vi "AccerlationAndSkidpadMonitoring.vi"() -> ()   [LabVIEW 2017]
uses:
  Control/AccelerationIndicator(Monitoring).ctl
  Control/SkidpadIndicator(Monitoring).ctl
  Control/AccelerationBestIndicator(Monitoring).ctl
  Control/AccerlationData.ctl
  Control/SkidpadData.ctl
panel:
  out "SkidpadBestIndicator":T1
  out "AccelerationBestIndicator":T1
  in  "Stop Button":bool
  out "SkidpadIndicator":T2
  out "AccelerationIndicator":T3
  # "2018 KSAE Formula Accerlation & Skidpad Event"
  # "Lap2 :"
  # "Lap4 :"
  # "Total :"
  # "Entry :"
  # "Univ. :"
  # "Time :"
  # "Entry :"
  # "Univ. :"
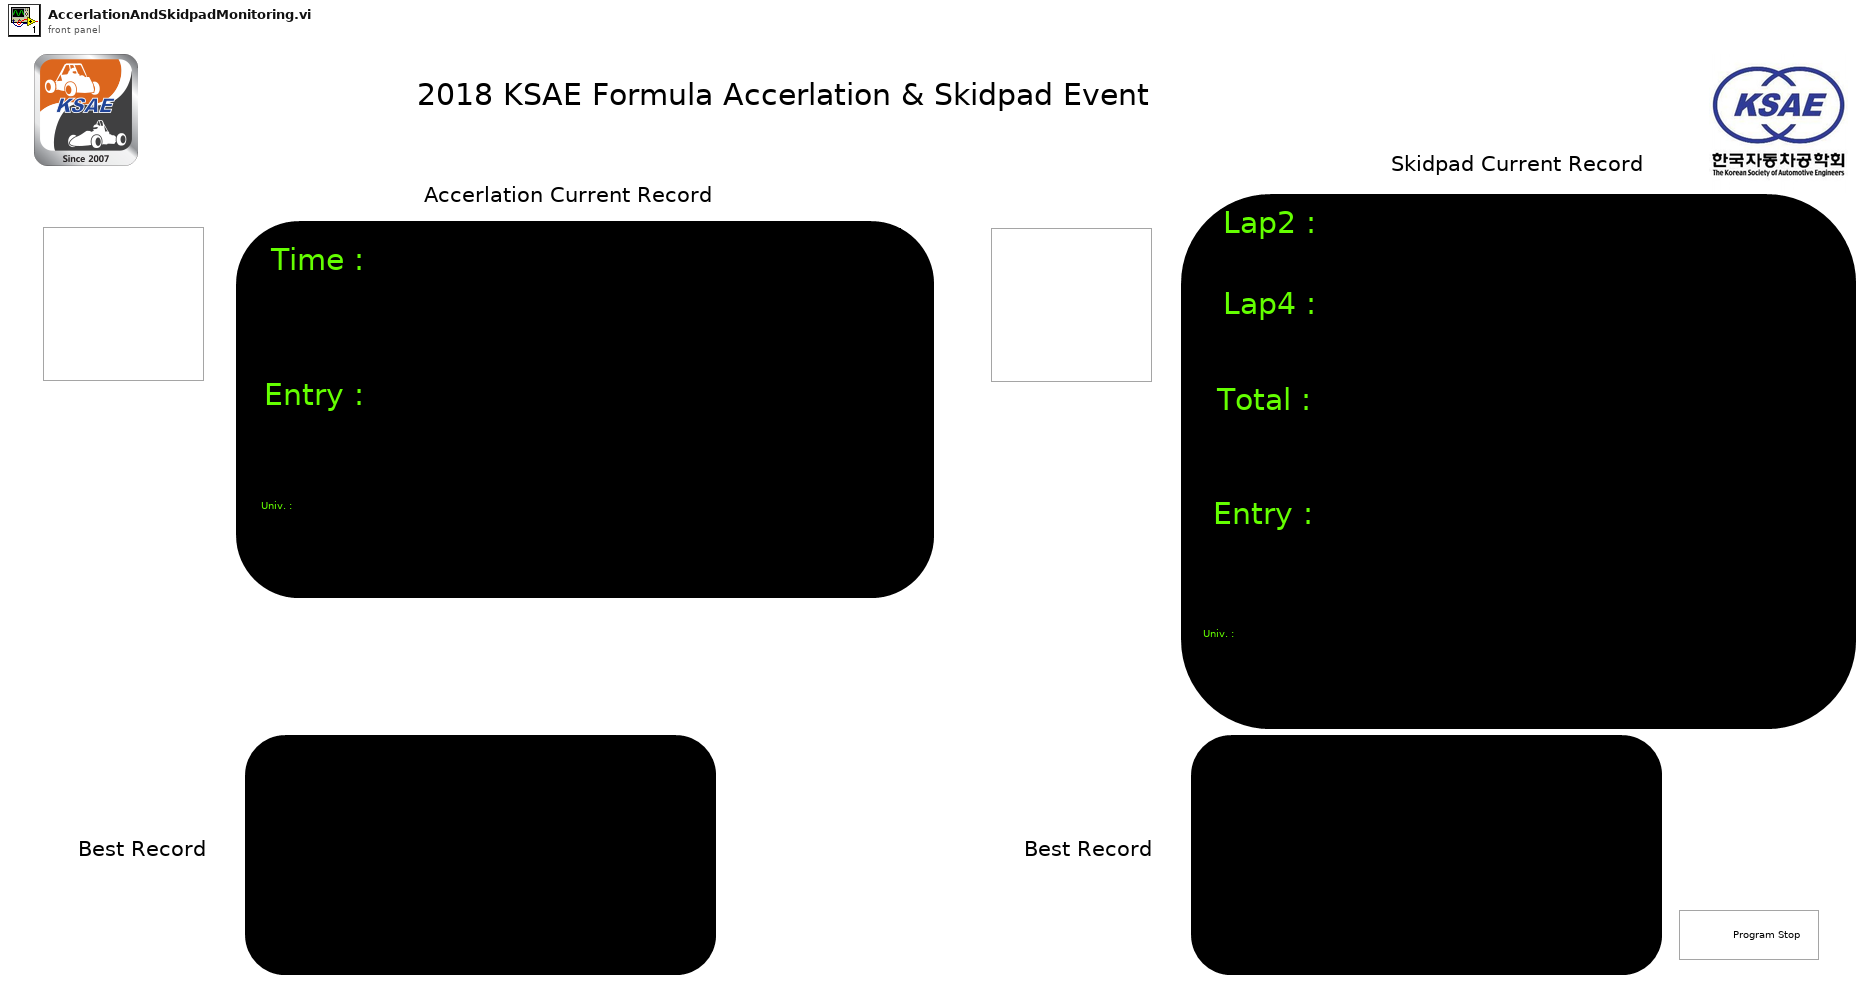
[diagram p1: front panel]
types:
  T1 = typedef "AccelerationBestIndicator(Monitoring).ctl" = cluster{"BestTime":string, "BestEntry":string, "BestSchool":string}
  T2 = typedef "SkidpadIndicator(Monitoring).ctl" = cluster{"Lab2":string, "Lab4":string, "TotalLabTime":string, "CurrentEntry":string, "CurrentSchool":string, "Flag":picture, "CurrentState":string}
  T3 = typedef "AccelerationIndicator(Monitoring).ctl" = cluster{"CurrentTime":string, "CurrentEntry":string, "CurrentUniversity":string, "Flag":picture, "CurrentState":string}
  T4 = typedef "SkidpadData.ctl" = cluster{"LabTime-2":string, "LabTime-4":string, "TotalLabTime":string, "Entry":string, "University":string, "Flag":picture, "Message":string, "TotalLabTimeBest":string, "EntryBest":string, "UniversityBest":string}
  T5 = cluster{"Read Access":enum8{"Allowed", "Required", "None"}, "Write Access":enum8{"Allowed", "Required", "None"}}
  T6 = typedef "AccerlationData.ctl" = cluster{"LabTimeCurrent":string, "EntryCurrent":string, "UniversityCurrent":string, "Flag":picture, "Message":string, "LabTimeBest":string, "EntryBest":string, "UniversityBest":string}
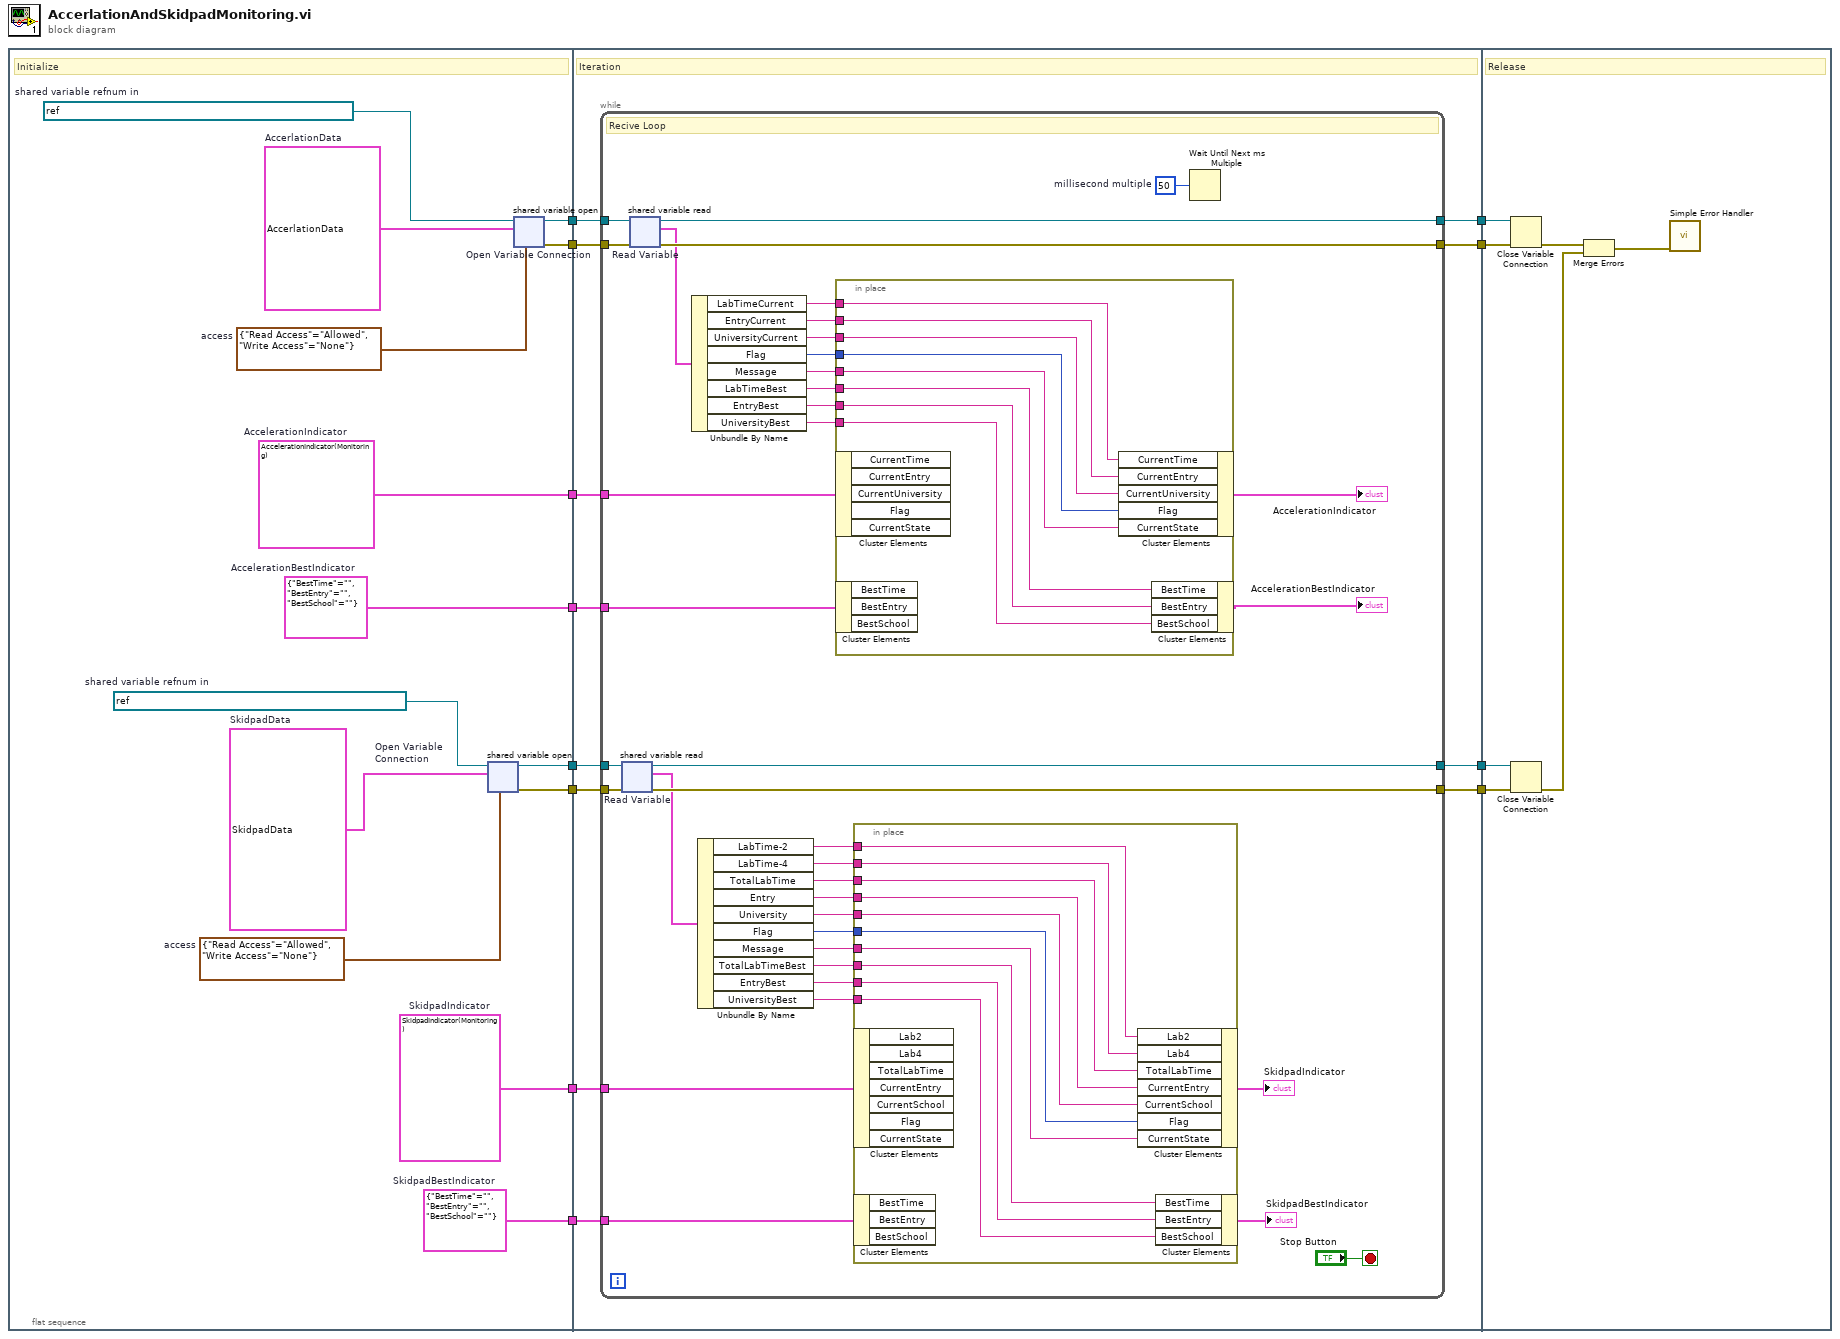
[diagram p0: block diagram]
diagram:
  n1 = flat-sequence {
    tunnel: [w25] -> w12
    tunnel: [w23] -> w11
    tunnel: [w20] -> w8
    tunnel: [w19] -> w7
    tunnel: [w17] -> w4
    tunnel: [w16] -> w3
    tunnel: [w15] -> w2
    tunnel: [w13] -> w1
    tunnel: w12 -> [w38]
    tunnel: w11 -> [w37]
    tunnel: [w36] -> w10
    tunnel: [w35] -> w9
    tunnel: w8 -> [w34]
    tunnel: w7 -> [w33]
    tunnel: [w32] -> w6
    tunnel: [w31] -> w5
    tunnel: w4 -> [w30]
    tunnel: w3 -> [w29]
    tunnel: w2 -> [w28]
    tunnel: w1 -> [w27]
    tunnel: w10 -> [w101]
    tunnel: w9 -> [w100]
    tunnel: w6 -> [w98]
    tunnel: w5 -> [w97]
    frame #0 {
      w13 = T1 {"BestTime"="", "BestEntry"="", "BestSchool"=""}  # SkidpadBestIndicator
      w14 = T4 {"LabTime-2"="", "LabTime-4"="", "TotalLabTime"="", "Entry"="", "University"="", "Flag"=bytes[0], "Message"="", "TotalLabTimeBest"="", "EntryBest"="", "UniversityBest"=""}  # SkidpadData
      w15 = T1 {"BestTime"="", "BestEntry"="", "BestSchool"=""}  # AccelerationBestIndicator
      w16 = T2 {"Lab2"="", "Lab4"="", "TotalLabTime"="", "CurrentEntry"="", "CurrentSchool"="", "Flag"=bytes[0], "CurrentState"=""}  # SkidpadIndicator
      w17 = T3 {"CurrentTime"="", "CurrentEntry"="", "CurrentUniversity"="", "Flag"=bytes[0], "CurrentState"=""}  # AccelerationIndicator
      w18 = refnum<k21> "ni.var.psp://kdh/MonitoringVariable/SkidpadData"  # shared variable refnum in
      w21 = T5 {"Read Access"=enum."Allowed", "Write Access"=enum."None"}  # access
      w22 = refnum<k21> "ni.var.psp://kdh/MonitoringVariable/AccerlationData"  # shared variable refnum in
      w24 = T5 {"Read Access"=enum."Allowed", "Write Access"=enum."None"}  # access
      w26 = T6 {"LabTimeCurrent"="", "EntryCurrent"="", "UniversityCurrent"="", "Flag"=bytes[0], "Message"="", "LabTimeBest"="", "EntryBest"="", "UniversityBest"=""}  # AccerlationData
      # "Initialize"
      n2 = shared-variable-open "Open Variable Connection"(w18, w14, w21) -> (w20:refnum<k21>, w19:errorcluster)  [unwired: 1 in]
      n3 = shared-variable-open "Open Variable Connection"(w22, w26, w24) -> (w25:refnum<k21>, w23:errorcluster)  [unwired: 1 in]
    }
    frame #1 {
      # "Iteration"
      n4 = while {
        tunnel: w38 -> [w76]
        tunnel: w37 -> [w75]
        tunnel: [w73] -> w35
        tunnel: [w72] -> w36
        tunnel: w34 -> [w70]
        tunnel: w33 -> [w69]
        tunnel: [w68] -> w32
        tunnel: [w67] -> w31
        tunnel: w30 -> [w65]
        tunnel: w29 -> [w58]
        tunnel: w28 -> [w48]
        tunnel: w27 -> [w43]
        stop <- "Stop Button" stop-if-true
        w74 = u32 50  # millisecond multiple
        # "Recive Loop"
        n5 = shared-variable-read "Read Variable"(w70, w69) -> (w68:refnum<k21>, w67:errorcluster, w66:T4)  [unwired: 1 out]
        n6 = shared-variable-read "Read Variable"(w76, w75) -> (w73:refnum<k21>, w72:errorcluster, w71:T6)  [unwired: 1 out]
        n7 = Unbundle By Name(w71) -> ("LabTimeCurrent"=w63:string, "EntryCurrent"=w62:string, "UniversityCurrent"=w61:string, "Flag"=w60:picture, "Message"=w59:string, "LabTimeBest"=w47:string, "EntryBest"=w46:string, "UniversityBest"=w45:string)
        n8 = Unbundle By Name(w66) -> ("LabTime-2"=w57:string, "LabTime-4"=w56:string, "TotalLabTime"=w55:string, "Entry"=w54:string, "University"=w52:string, "Flag"=w51:picture, "Message"=w50:string, "TotalLabTimeBest"=w42:string, "EntryBest"=w41:string, "UniversityBest"=w40:string)
        n9 = in-place {
          in-place-border: w63 -> [w94]
          in-place-border: w62 -> [w93]
          in-place-border: w61 -> [w92]
          in-place-border: w60 -> [w91]
          in-place-border: w59 -> [w90]
          in-place-border: w47 -> [w89]
          in-place-border: w46 -> [w88]
          in-place-border: w45 -> [w87]
          n10 = in-place-cluster #1(w65) -> ()  [unwired: 5 out]
          n11 = in-place-cluster #2(w48) -> ()  [unwired: 3 out]
          n12 = in-place-cluster #1("CurrentTime"=w94, "CurrentEntry"=w93, "CurrentUniversity"=w92, "Flag"=w91, "CurrentState"=w90) -> (→"AccelerationIndicator":T3)
          n13 = in-place-cluster #2("BestTime"=w89, "BestEntry"=w88, "BestSchool"=w87) -> (→"AccelerationBestIndicator":T1)
        }
        n14 = in-place {
          in-place-border: w57 -> [w86]
          in-place-border: w56 -> [w85]
          in-place-border: w55 -> [w84]
          in-place-border: w54 -> [w83]
          in-place-border: w52 -> [w82]
          in-place-border: w51 -> [w81]
          in-place-border: w50 -> [w80]
          in-place-border: w42 -> [w79]
          in-place-border: w41 -> [w78]
          in-place-border: w40 -> [w77]
          n15 = in-place-cluster #3(w58) -> ()  [unwired: 7 out]
          n16 = in-place-cluster #4(w43) -> ()  [unwired: 3 out]
          n17 = in-place-cluster #3("Lab2"=w86, "Lab4"=w85, "TotalLabTime"=w84, "CurrentEntry"=w83, "CurrentSchool"=w82, "Flag"=w81, "CurrentState"=w80) -> (→"SkidpadIndicator":T2)
          n18 = in-place-cluster #4("BestTime"=w79, "BestEntry"=w78, "BestSchool"=w77) -> (→"SkidpadBestIndicator":T1)
        }
        n19 = Wait Until Next ms Multiple(millisecond multiple=w74) -> ()  [unwired: 1 out]
      }
    }
    frame #2 {
      # "Release"
      n20 = Close Variable Connection(8:w101, 11:w100) -> (0:w99:errorcluster)
      n21 = Close Variable Connection(8:w97, 11:w98) -> (0:w95:errorcluster)
      n22 = Merge Errors "Merge Errors"(w99, w95) -> (w96:errorcluster)
      n23 = call <vilib>:"Simple Error Handler.vi"("error in (no error)"=w96) -> ()  [unwired: 4 in, 5 out]
    }
  }
